vi "基础20.vi"() -> ()   [LabVIEW 2014]
panel:
  out "字符串":string
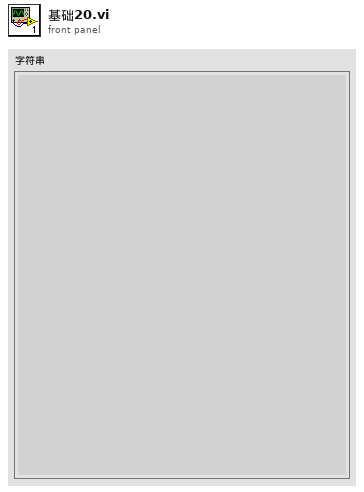
[diagram p1: front panel]
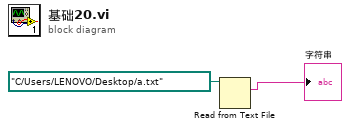
[diagram p0: block diagram]
diagram:
  n1 = Read from Text File(file (use dialog)=path "C:/Users/LENOVO/Desktop/a.txt" ("文件（使用对话框）")) -> (text=→"字符串":string)  [unwired: 3 in, 3 out]
